vi "02_Search_SplitString.vi"(11 "String":string) -> (3 "count":i32)   [LabVIEW 2020, in "client.lvclass"]
uses:
  client.lvclass
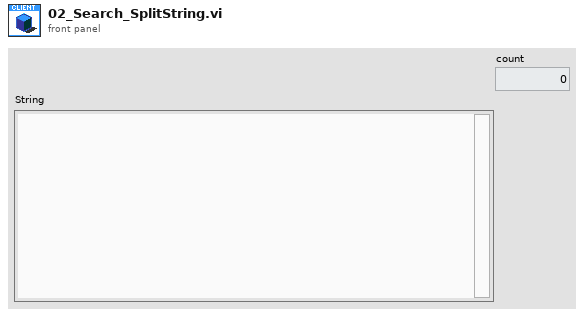
[diagram p1: front panel]
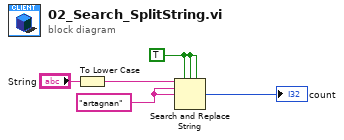
[diagram p0: block diagram]
diagram:
  w2 = TRUE ("replace all? (F)")
  w1 = "artagnan"
  n1 = To Lower Case(string="String") -> (all lower case string=w4:string)
  n2 = Search and Replace String(replace all?=w2, case sensitive?=w2, multiline?=w2, input string=w4, search string=w1, replace string=w1) -> (number of replacements=→"count":i32)  [unwired: 2 in, 3 out]
